vi "x-axis.vi"(8 "error in (no error)":errorcluster, 11 "Function Gen Scan in":refnum<class "Function Gen Scan.lvclass">) -> (0 "error out":errorcluster, 1 "Label":string, 2 "Unit":string, 3 "Function Gen Scan out":refnum<class "Function Gen Scan.lvclass">)   [LabVIEW 2017, in "Function Gen Scan.lvclass"]
uses:
  Function Gen Scan.lvclass
  Scanner/Scanner.lvclass
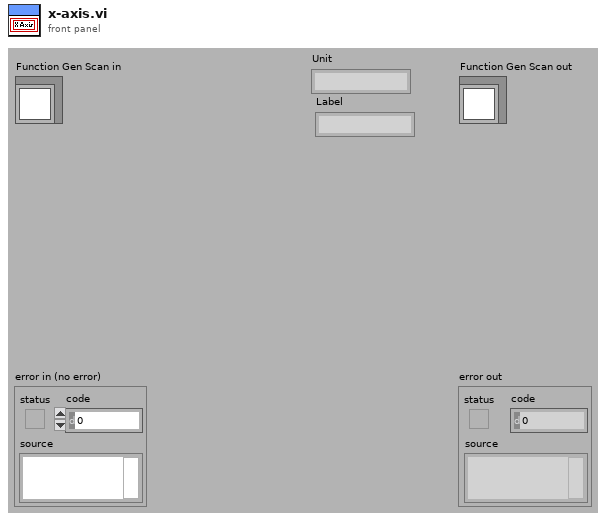
[diagram p1: front panel]
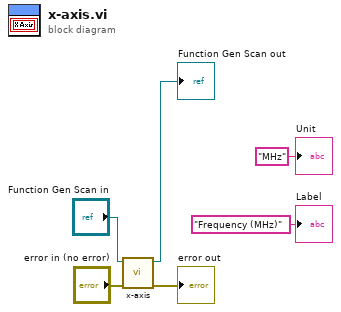
[diagram p0: block diagram]
diagram:
  n1 = call-parent "x-axis.vi"("error in (no error)"="error in (no error)", "Scanner in"="Function Gen Scan in") -> ("error out"=→"error out":errorcluster, "Scanner out"=→"Function Gen Scan out":refnum<class "Function Gen Scan.lvclass">)  [unwired: 6 in, 2 out]
  "Label" <- "Frequency (MHz)" ("Label")
  "Unit" <- "MHz" ("Unit")
